vi "SNRStructure.vi"(8 "Digitizer Analyze Input":T1={"Pins"=["Xout"], "Published Data Id"=[], "frequency range"={"start frequency"=-1.0, "stop frequency"=-1.0}}, 9 "RFSG Input":T3={"LO configure setting"={"Carrier Frequency (Hz)"=5180000000.0, "Power Level(dBm)"=-10.0, "External Attenuation (dB)"=0.0}, "Port"=""} {"LO configure setting"."Carrier Frequency (Hz)" format="%#_6p"}, 10 "Scope Input":T2={"Min. Sample Rate"=0.0, "Min Record Length"=0, "Vertical Coupling"=1, "Vertical Range (V)"=2.0, "Pins"=["Xout"]} {"Vertical Range (V)" format="%_3g"; "Vertical Coupling" items=["AC", "DC", "Ground"]; "Min. Sample Rate" format="%#_6p"}, 11 "Semiconductor Module Context":T4) -> (0 "error out":errorcluster)   [LabVIEW 2014]
uses:
  <vilib>/NI_TestStand_SemiconductorModule/NI_TestStand_Semiconductor_Module.lvlibp/PinMap/General/SemiconductorModuleContext.ctl
  Control/RFSG Input.ctl
  Control/Scope Input.ctl
  Control/Digitizier Analyze Input.ctl
  Control/Quene Type_Digitizer.ctl
  <vilib>/NI_TestStand_SemiconductorModule/NI_TestStand_Semiconductor_Module.lvlibp/PinMap/RF/RFPM/PinToNIRFPMSessions.vi
  <vilib>/NI_TestStand_SemiconductorModule/NI_TestStand_Semiconductor_Module.lvlibp
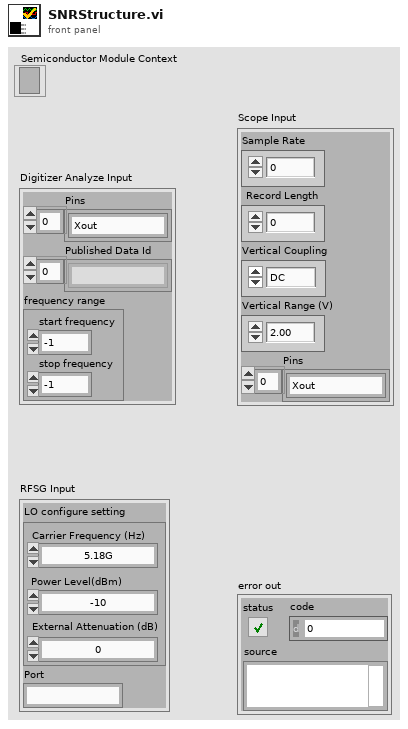
[diagram p1: front panel]
types:
  T1 = typedef "Digitizier Analyze Input.ctl" = cluster{"Pins":string[], "Published Data Id":string[], "frequency range":cluster{"start frequency":dbl, "stop frequency":dbl}}
  T2 = typedef "Scope Input.ctl" = cluster{"Min. Sample Rate":dbl, "Min Record Length":i32, "Vertical Coupling":i32, "Vertical Range (V)":dbl, "Pins":string[]}
  T3 = typedef "RFSG Input.ctl" = cluster{"LO configure setting":cluster{"Carrier Frequency (Hz)":dbl, "Power Level(dBm)":dbl, "External Attenuation (dB)":dbl}, "Port":string}
  T4 = typedef "NI_TestStand_Semiconductor_Module.lvlibp/SemiconductorModuleContext.ctl" = refnum<k7>
  T5 = typedef "Quene Type_Digitizer.ctl" = cluster{"Actiion":enum16{"Exit", "Analyze"}, "Waveform Data":waveform(dbl)[], "Semiconductor Module Context":T4, "error constant":errorcluster}
  T6 = cluster{"Carrier Frequency (Hz)":dbl, "Power Level(dBm)":dbl, "External Attenuation (dB)":dbl}
  T7 = cluster{"start frequency":dbl, "stop frequency":dbl}
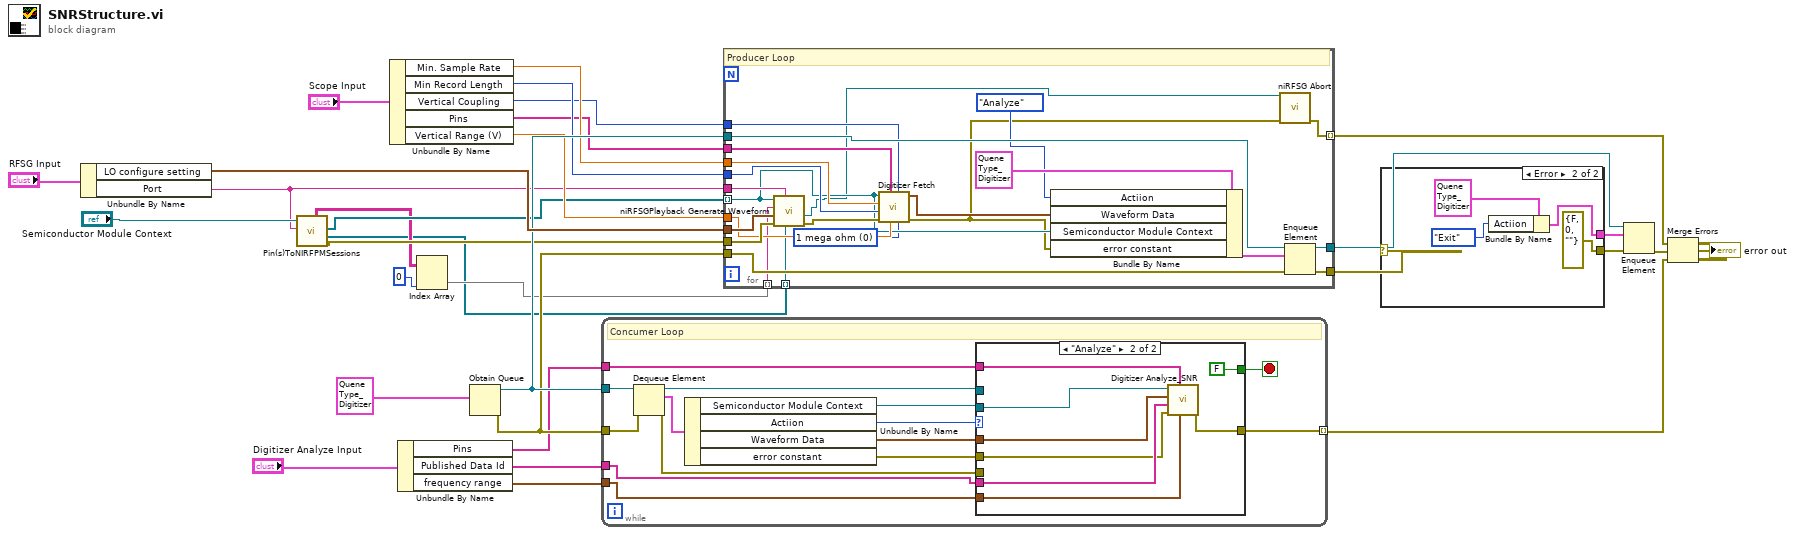
[diagram p0: block diagram]
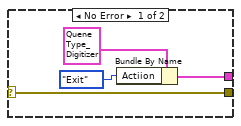
[diagram p2: hidden frame]
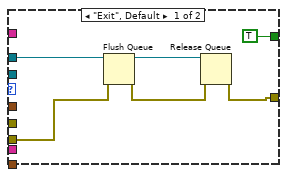
[diagram p3: hidden frame]
diagram:
  n1 = Unbundle By Name("RFSG Input") -> ("LO configure setting"=w29:T6, "Port"=w8:string)
  n2 = call-poly <vilib>:"Pin(s)ToNIRFPMSessions.vi"("Pin"=w8, "Semiconductor Module Context"="Semiconductor Module Context") -> ("error out"=w6:errorcluster, "Instrument Sessions"=w2:refnum<k15>[], "Semiconductor Module Contexts"=w7:refnum<k7>[], "Ports List"=w4:string[][])  [unwired: 4 in, 2 out]
  n3 = Unbundle By Name("Scope Input") -> ("Min. Sample Rate"=w17:dbl, "Min Record Length"=w18:i32, "Vertical Coupling"=w16:i32, "Pins"=w11:string[], "Vertical Range (V)"=w10:dbl)
  n4 = Unbundle By Name("Digitizer Analyze Input") -> ("Pins"=w13:string[], "Published Data Id"=w14:string[], "frequency range"=w12:T7)
  n5 = Index Array(array=w4, index (col)=0) -> (element=w3:string[])  [unwired: 1 in]
  n6 = Obtain Queue(element data type=T5 {"Actiion"=enum."Analyze", "Waveform Data"=[], "Semiconductor Module Context"=refnum, "error constant"={"status"=FALSE, "code"=0, "source"=""}}) -> (queue out=w27:refnum<queue>, error out=w22:errorcluster)  [unwired: 4 in, 1 out]
  n7 = while {
    tunnel: w27 -> [w45]
    tunnel: w14 -> [w39]
    tunnel: w13 -> [w38]
    tunnel: w22 -> [w44]
    tunnel: [w35] -> w24 mode=indexing
    tunnel: w12 -> [w34]
    stop <- w41 stop-if-true
    # "Concumer Loop"
    n8 = Dequeue Element(queue=w45, error in (no error)=w44) -> (queue out=w37:refnum<queue>, element=w43:T5, error out=w36:errorcluster)  [unwired: 1 in, 1 out]
    n9 = Unbundle By Name(w43) -> ("Semiconductor Module Context"=w33:T4, "Actiion"=w42:enum16{"Exit", "Analyze"}, "Waveform Data"=w40:waveform(dbl)[], "error constant"=w32:errorcluster)
    n10 = case shown="\"Analyze\"" w42 {
      tunnel: [TRUE FALSE] -> w41
      tunnel: w33 -> [_ w55]
      tunnel: w40 -> [_ w58]
      tunnel: w39 -> [_ w56]
      tunnel: w38 -> [_ w54]
      tunnel: w37 -> [w48 _]
      tunnel: w36 -> [w47 _]
      tunnel: [w46 w57] -> w35
      tunnel: w34 -> [_ w53]
      tunnel: w32 -> [_ w52]
      frame "Exit", Default {
        n11 = Flush Queue(queue=w48, error in (no error)=w47) -> (queue out=w50:refnum<queue>, error out=w49:errorcluster)  [unwired: 1 out]
        n12 = Release Queue(queue=w50, error in (no error)=w49) -> (error out=w46:errorcluster)  [unwired: 1 in, 2 out]
      }
      frame "Analyze" {
        n13 = call "Digitizer Analyze_SNR.vi"("frequency range"=w53, "Pins"=w54, "error in"=w52, "Published Data Id"=w56, "Waveform Data In"=w58, "Semiconductor Module Context"=w55) -> ("error out"=w57:errorcluster)  [unwired: 2 in, 3 out]
      }
    }
  }
  n14 = for {
    tunnel: w7 -> [w64] mode=indexing
    tunnel: w29 -> [w82]
    tunnel: w8 -> [w81]
    tunnel: w27 -> [w80]
    tunnel: [w74] -> w28
    tunnel: w6 -> [w83]
    tunnel: [w62] -> w23 mode=indexing
    tunnel: w22 -> [w73]
    tunnel: [w75] -> w21
    tunnel: w18 -> [w68]
    tunnel: w17 -> [w71]
    tunnel: w16 -> [w69]
    tunnel: w11 -> [w72]
    tunnel: w10 -> [w67]
    tunnel: w3 -> [w66] mode=indexing
    tunnel: w2 -> [w65] mode=indexing
    w61 = u32 0 items=["1 mega ohm"=0, "50 ohms"=2] ("input impedance")
    # "Producer Loop"
    n15 = call "niRFSGPlayback Generate Waveform.vi"("instrument handle"=w65, "Port"=w81, "error in (no error)"=w83, "LO configure setting"=w82, "TX port"=w66, "TSM Context"=w64) -> ("error out"=w70:errorcluster, "instrument handle out"=w63:refnum<k15>)  [unwired: 4 in]
    n16 = call "Digitizer Fetch.vi"("input impedance"=w61, "Vertical Coupling"=w69, "Vertical Range (V)"=w67, "Pins"=w72, "error in (no error)"=w70, "Min Record Length"=w68, "Min. Sample Rate"=w71, "Semiconductor Module Context"=w64) -> ("error out"=w60:errorcluster, "Waveform Data Out"=w78:waveform(dbl)[])  [unwired: 2 in]
    n17 = Bundle By Name(cluster=T5 {"Actiion"=enum."Exit", "Waveform Data"=[], "Semiconductor Module Context"=refnum, "error constant"={"status"=FALSE, "code"=0, "source"=""}}, "Actiion"=enum16{"Exit", "Analyze"}."Analyze", "Waveform Data"=w78, "Semiconductor Module Context"=w64, "error constant"=w60) -> (w76:T5)
    n18 = call <instrlib>:"niRFSG Abort.vi"("instrument handle"=w63, "error in"=w60) -> ("error out"=w62:errorcluster)  [unwired: 12 in, 1 out]
    n19 = Enqueue Element(queue=w80, element=w76, error in (no error)=w73) -> (queue out=w74:refnum<queue>, error out=w75:errorcluster)  [unwired: 1 in, 1 out]
  }
  n20 = case shown="Error" w21 {
    selector: w21 -> [w85 _]
    tunnel: [w86 w89] -> w1
    tunnel: [w85 errorcluster {"status"=FALSE, "code"=0, "source"=""} ("error IO")] -> w20
    frame No Error {
      n21 = Bundle By Name(cluster=T5 {"Actiion"=enum."Exit", "Waveform Data"=[], "Semiconductor Module Context"=refnum, "error constant"={"status"=FALSE, "code"=0, "source"=""}}, "Actiion"=enum16{"Exit", "Analyze"}."Exit") -> (w86:T5)
    }
    frame Error {
      n22 = Bundle By Name(cluster=T5 {"Actiion"=enum."Exit", "Waveform Data"=[], "Semiconductor Module Context"=refnum, "error constant"={"status"=FALSE, "code"=0, "source"=""}}, "Actiion"=enum16{"Exit", "Analyze"}."Exit") -> (w89:T5)
    }
  }
  n23 = Enqueue Element(queue=w28, element=w1, error in (no error)=w20) -> (error out=w25:errorcluster)  [unwired: 1 in, 2 out]
  n24 = Merge Errors(w23, w25, w24) -> (→"error out":errorcluster)
